vi "AudibleAlarm.vi"   [LabVIEW 2012]
uses:
  <vilib>/measure/NI_MABase.lvlib
types:
  T1 = cluster{"frequency":dbl, "amplitude":dbl, "phase":dbl}[]
  T2 = cluster{"frequency":dbl, "amplitude":dbl, "phase":dbl}
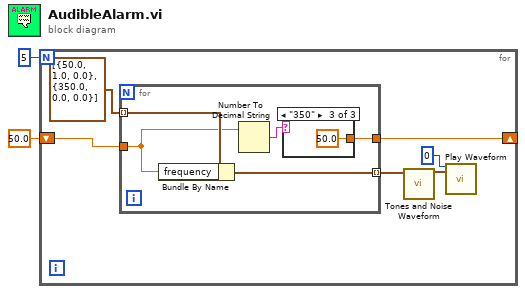
[diagram p0: block diagram]
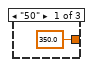
[diagram p2: hidden frame]
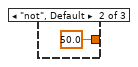
[diagram p3: hidden frame]
diagram:
  n1 = for {
    N: 5 -> [_]
    shift-right: [w3] -> _
    shift-left: 50.0 ("frequency") -> [w4]
    n2 = for {
      tunnel: T1 [{"frequency"=50.0, "amplitude"=1.0, "phase"=0.0}, {"frequency"=350.0, "amplitude"=0.0, "phase"=0.0}] ("tones") -> [w13] mode=indexing
      tunnel: [w12] -> w5 mode=indexing
      tunnel: w4 -> [w10]
      tunnel: [w9] -> w3
      n3 = Bundle By Name(cluster=w13, "frequency"=w10) -> (w12:T2)
      n4 = Number To Decimal String(number=w10) -> (decimal integer string=w11:string)  [unwired: 1 in]
      n5 = case shown="\"350\"" w11 {
        tunnel: [350.0 ("frequency") 50.0 ("frequency") 50.0 ("frequency")] -> w9
        frame "50" {
        }
        frame "not", Default {
        }
        frame "350" {
        }
      }
    }
    n6 = call <vilib>:"Tones and Noise Waveform.vi"("tones"=w5) -> ("signal out"=w7:waveform(dbl))  [unwired: 9 in, 1 out]
    n7 = call "Play Waveform"("Device"=u32 0, "Data"=w7) -> ()  [unwired: 17 in, 1 out]
  }
